vi "Blue to yellow 3.vi"   [LabVIEW 2019]
uses:
  Global Var.vi
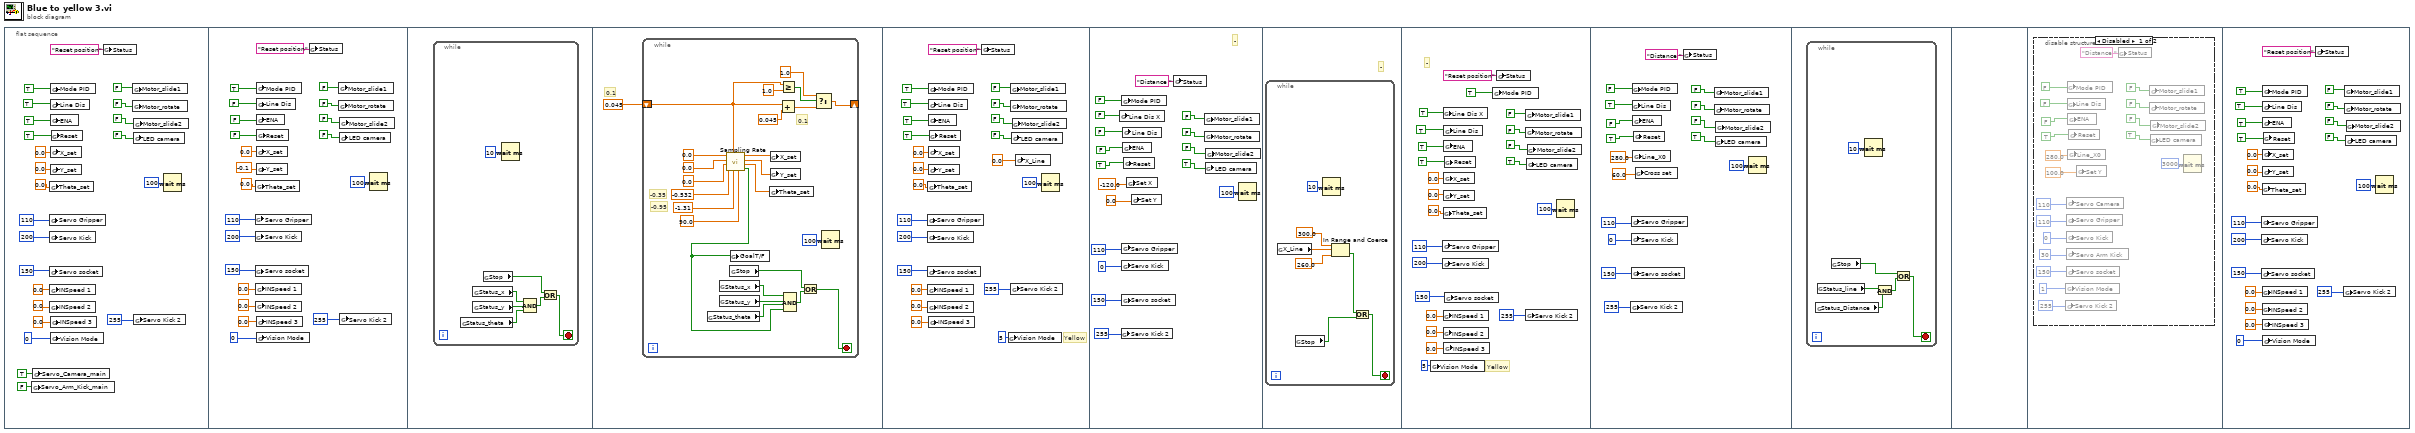
[diagram p0: block diagram]
diagram:
  n1 = flat-sequence {
    frame #0 {
      n2 = global write "Global Var.vi" "Servo_Arm_Kick_main"(FALSE ("Mode PID")) -> ()
      n3 = global write "Global Var.vi" "Servo_Camera_main"(TRUE ("Mode PID")) -> ()
      n4 = global write "Global Var.vi" "Servo Gripper"(u8 110 ("Servo Camera")) -> ()
      n5 = global write "Global Var.vi" "Servo Kick"(u8 200 ("Servo Camera")) -> ()
      n6 = global write "Global Var.vi" "Servo socket"(u8 150 ("Servo Camera")) -> ()
      n7 = global write "Global Var.vi" "Theta_set"(0.0 ("Theta_set")) -> ()
      n8 = global write "Global Var.vi" "INSpeed 1"(0.0 ("X_set")) -> ()
      n9 = global write "Global Var.vi" "INSpeed 2"(0.0 ("Y_set")) -> ()
      n10 = global write "Global Var.vi" "Mode PID"(TRUE ("Mode PID")) -> ()
      n11 = global write "Global Var.vi" "Line Dis"(TRUE ("Mode PID")) -> ()
      n12 = global write "Global Var.vi" "ENA"(TRUE ("ENA")) -> ()
      n13 = global write "Global Var.vi" "X_set"(0.0 ("X_set")) -> ()
      n14 = global write "Global Var.vi" "Y_set"(0.0 ("Y_set")) -> ()
      n15 = global write "Global Var.vi" "INSpeed 3"(0.0 ("Theta_set")) -> ()
      n16 = global write "Global Var.vi" "Vision Mode"(i16 0 ("Vision Mode")) -> ()
      n17 = global write "Global Var.vi" "Reset"(TRUE ("ENA")) -> ()
      n18 = global write "Global Var.vi" "Status"("Reset position" ("Status")) -> ()
      n19 = global write "Global Var.vi" "Motor_slide1"(FALSE ("Mode PID")) -> ()
      n20 = global write "Global Var.vi" "Motor_rotate"(FALSE ("ENA")) -> ()
      n21 = global write "Global Var.vi" "LED camera"(FALSE ("LED camera")) -> ()
      n22 = global write "Global Var.vi" "Motor_slide2"(FALSE ("ENA")) -> ()
      n23 = global write "Global Var.vi" "Servo Kick 2"(u8 255 ("Servo Camera")) -> ()
      n24 = Wait (ms)(milliseconds to wait=u32 100) -> ()  [unwired: 1 out]
    }
    frame #1 {
      n25 = global write "Global Var.vi" "Servo Gripper"(u8 110 ("Servo Camera")) -> ()
      n26 = global write "Global Var.vi" "Servo Kick"(u8 200 ("Servo Camera")) -> ()
      n27 = global write "Global Var.vi" "Servo socket"(u8 150 ("Servo Camera")) -> ()
      n28 = global write "Global Var.vi" "Theta_set"(0.0 ("Theta_set")) -> ()
      n29 = global write "Global Var.vi" "INSpeed 1"(0.0 ("X_set")) -> ()
      n30 = global write "Global Var.vi" "INSpeed 2"(0.0 ("Y_set")) -> ()
      n31 = global write "Global Var.vi" "Mode PID"(TRUE ("Mode PID")) -> ()
      n32 = global write "Global Var.vi" "Line Dis"(FALSE ("Mode PID")) -> ()
      n33 = global write "Global Var.vi" "ENA"(FALSE ("ENA")) -> ()
      n34 = global write "Global Var.vi" "X_set"(0.0 ("X_set")) -> ()
      n35 = global write "Global Var.vi" "Y_set"(-0.1 ("Y_set")) -> ()
      n36 = global write "Global Var.vi" "INSpeed 3"(0.0 ("Theta_set")) -> ()
      n37 = global write "Global Var.vi" "Vision Mode"(i16 0 ("Vision Mode")) -> ()
      n38 = global write "Global Var.vi" "Reset"(FALSE ("ENA")) -> ()
      n39 = global write "Global Var.vi" "Status"("Reset position" ("Status")) -> ()
      n40 = global write "Global Var.vi" "Motor_slide1"(FALSE ("Mode PID")) -> ()
      n41 = global write "Global Var.vi" "Motor_rotate"(FALSE ("ENA")) -> ()
      n42 = global write "Global Var.vi" "LED camera"(FALSE ("LED camera")) -> ()
      n43 = global write "Global Var.vi" "Motor_slide2"(FALSE ("ENA")) -> ()
      n44 = global write "Global Var.vi" "Servo Kick 2"(u8 255 ("Servo Camera")) -> ()
      n45 = Wait (ms)(milliseconds to wait=u32 100) -> ()  [unwired: 1 out]
    }
    frame #2 {
      n46 = while {
        stop <- w47 stop-if-true
        n47 = global read "Global Var.vi" "Status_theta"() -> (w49:bool)
        n48 = global read "Global Var.vi" "Status_x"() -> (w50:bool)
        n49 = global read "Global Var.vi" "Status_y"() -> (w51:bool)
        n50 = global read "Global Var.vi" "Stop"() -> (w45:bool)
        n51 = Wait (ms)(milliseconds to wait=u32 10) -> ()  [unwired: 1 out]
        n52 = Compound Arithmetic op=AND(w50, w51, w49) -> (w46:bool)
        n53 = Or(x=w45, y=w46) -> (x .or. y?=w47:bool)
      }
    }
    frame #3 {
      # "0.1"
      n54 = while {
        shift-right: [w55] -> _
        shift-left: 0.045 -> [w53]
        stop <- w72 stop-if-true
        # "0.1"
        # "-0.95"
        # "-0.35"
        n55 = global read "Global Var.vi" "Status_theta"() -> (w74:bool)
        n56 = global read "Global Var.vi" "Status_x"() -> (w75:bool)
        n57 = global read "Global Var.vi" "Status_y"() -> (w76:bool)
        n58 = call "Sampling Rate.vi"("input a1"=90.0, "input y1"=-1.31, "T(0-1)"=w53, "input x1"=-0.532, "input a0"=0.0, "input y0"=0.0, "input x0"=0.0) -> ("GoalT/F"=w60:bool, "a_output"=w67:dbl, "y_output"=w68:dbl, "x_output"=w69:dbl)  [unwired: 1 in]
        n59 = global read "Global Var.vi" "Stop"() -> (w70:bool)
        n60 = global write "Global Var.vi" "GoalT/F"(w60) -> ()
        n61 = global write "Global Var.vi" "Theta_set"(w67) -> ()
        n62 = global write "Global Var.vi" "X_set"(w69) -> ()
        n63 = global write "Global Var.vi" "Y_set"(w68) -> ()
        n64 = Add(x=w53, y=0.045) -> (x+y=w58:dbl)
        n65 = Greater Or Equal?(x=w53, y=1.0) -> (x >= y?=w57:bool)
        n66 = Compound Arithmetic op=AND(w75, w76, w74, w60) -> (w71:bool)
        n67 = Or(x=w70, y=w71) -> (x .or. y?=w72:bool)
        n68 = Select(t=1.0, s=w57, f=w58) -> (s? t:f=w55:dbl)
        n69 = Wait (ms)(milliseconds to wait=u32 100) -> ()  [unwired: 1 out]
      }
    }
    frame #4 {
      # "Yellow"
      n70 = global write "Global Var.vi" "Servo Gripper"(u8 110 ("Servo Camera")) -> ()
      n71 = global write "Global Var.vi" "Servo Kick"(u8 200 ("Servo Camera")) -> ()
      n72 = global write "Global Var.vi" "Servo socket"(u8 150 ("Servo Camera")) -> ()
      n73 = global write "Global Var.vi" "Theta_set"(0.0 ("Theta_set")) -> ()
      n74 = global write "Global Var.vi" "INSpeed 1"(0.0 ("X_set")) -> ()
      n75 = global write "Global Var.vi" "INSpeed 2"(0.0 ("Y_set")) -> ()
      n76 = global write "Global Var.vi" "Mode PID"(TRUE ("Mode PID")) -> ()
      n77 = global write "Global Var.vi" "Line Dis"(TRUE ("Mode PID")) -> ()
      n78 = global write "Global Var.vi" "ENA"(TRUE ("ENA")) -> ()
      n79 = global write "Global Var.vi" "X_set"(0.0 ("X_set")) -> ()
      n80 = global write "Global Var.vi" "Y_set"(0.0 ("Y_set")) -> ()
      n81 = global write "Global Var.vi" "INSpeed 3"(0.0 ("Theta_set")) -> ()
      n82 = global write "Global Var.vi" "Reset"(TRUE ("ENA")) -> ()
      n83 = global write "Global Var.vi" "Status"("Reset position" ("Status")) -> ()
      n84 = global write "Global Var.vi" "Vision Mode"(i16 5 ("Vision Mode")) -> ()
      n85 = global write "Global Var.vi" "Motor_slide1"(FALSE ("Mode PID")) -> ()
      n86 = global write "Global Var.vi" "Motor_rotate"(FALSE ("ENA")) -> ()
      n87 = global write "Global Var.vi" "Servo Kick 2"(u8 255 ("Servo Camera")) -> ()
      n88 = global write "Global Var.vi" "LED camera"(FALSE ("LED camera")) -> ()
      n89 = global write "Global Var.vi" "Motor_slide2"(FALSE ("ENA")) -> ()
      n90 = global write "Global Var.vi" "X_Line"(0.0 ("X_set")) -> ()
      n91 = Wait (ms)(milliseconds to wait=u32 100) -> ()  [unwired: 1 out]
    }
    frame #5 {
      # "-"
      n92 = global write "Global Var.vi" "Line Dis X"(FALSE ("Mode PID")) -> ()
      n93 = global write "Global Var.vi" "Servo Kick 2"(u8 255 ("Servo Camera")) -> ()
      n94 = global write "Global Var.vi" "Mode PID"(FALSE ("Mode PID")) -> ()
      n95 = global write "Global Var.vi" "Servo Gripper"(u8 110 ("Servo Camera")) -> ()
      n96 = global write "Global Var.vi" "Servo Kick"(u8 0 ("Servo Camera")) -> ()
      n97 = global write "Global Var.vi" "Servo socket"(u8 150 ("Servo Camera")) -> ()
      n98 = global write "Global Var.vi" "Line Dis"(FALSE ("Mode PID")) -> ()
      n99 = global write "Global Var.vi" "ENA"(FALSE ("ENA")) -> ()
      n100 = global write "Global Var.vi" "Reset"(TRUE ("ENA")) -> ()
      n101 = global write "Global Var.vi" "Set X"(-120.0 ("Y_set")) -> ()
      n102 = global write "Global Var.vi" "Set Y"(0.0 ("Y_set")) -> ()
      n103 = global write "Global Var.vi" "Status"("Distance " ("Status")) -> ()
      n104 = global write "Global Var.vi" "Motor_slide1"(FALSE ("Mode PID")) -> ()
      n105 = global write "Global Var.vi" "Motor_rotate"(FALSE ("ENA")) -> ()
      n106 = global write "Global Var.vi" "LED camera"(TRUE ("LED camera")) -> ()
      n107 = global write "Global Var.vi" "Motor_slide2"(FALSE ("ENA")) -> ()
      n108 = Wait (ms)(milliseconds to wait=u32 100) -> ()  [unwired: 1 out]
    }
    frame #6 {
      # "-"
      n109 = while {
        stop <- w121 stop-if-true
        n110 = global read "Global Var.vi" "X_Line"() -> (w119:dbl)
        n111 = global read "Global Var.vi" "Stop"() -> (w120:bool)
        n112 = Wait (ms)(milliseconds to wait=u32 10) -> ()  [unwired: 1 out]
        n113 = In Range and Coerce(upper limit=300.0, x=w119, lower limit=260.0) -> (In Range?=w116:bool)  [unwired: 1 out]
        n114 = Or(x=w116, y=w120) -> (x .or. y?=w121:bool)
      }
    }
    frame #7 {
      # "-"
      # "Yellow"
      n115 = global write "Global Var.vi" "Vision Mode"(i16 5 ("Vision Mode")) -> ()
      n116 = global write "Global Var.vi" "Servo Gripper"(u8 110 ("Servo Camera")) -> ()
      n117 = global write "Global Var.vi" "Servo Kick"(u8 200 ("Servo Camera")) -> ()
      n118 = global write "Global Var.vi" "Line Dis X"(TRUE ("Mode PID")) -> ()
      n119 = global write "Global Var.vi" "Theta_set"(0.0 ("Theta_set")) -> ()
      n120 = global write "Global Var.vi" "INSpeed 1"(0.0 ("X_set")) -> ()
      n121 = global write "Global Var.vi" "INSpeed 2"(0.0 ("Y_set")) -> ()
      n122 = global write "Global Var.vi" "Line Dis"(TRUE ("Mode PID")) -> ()
      n123 = global write "Global Var.vi" "ENA"(TRUE ("ENA")) -> ()
      n124 = global write "Global Var.vi" "X_set"(0.0 ("X_set")) -> ()
      n125 = global write "Global Var.vi" "Y_set"(0.0 ("Y_set")) -> ()
      n126 = global write "Global Var.vi" "INSpeed 3"(0.0 ("Theta_set")) -> ()
      n127 = global write "Global Var.vi" "Reset"(TRUE ("ENA")) -> ()
      n128 = global write "Global Var.vi" "Servo socket"(u8 150 ("Servo Camera")) -> ()
      n129 = global write "Global Var.vi" "Mode PID"(TRUE ("Mode PID")) -> ()
      n130 = global write "Global Var.vi" "Status"("Reset position" ("Status")) -> ()
      n131 = global write "Global Var.vi" "Motor_slide1"(FALSE ("Mode PID")) -> ()
      n132 = global write "Global Var.vi" "Motor_rotate"(FALSE ("ENA")) -> ()
      n133 = global write "Global Var.vi" "Servo Kick 2"(u8 255 ("Servo Camera")) -> ()
      n134 = global write "Global Var.vi" "LED camera"(TRUE ("LED camera")) -> ()
      n135 = global write "Global Var.vi" "Motor_slide2"(FALSE ("ENA")) -> ()
      n136 = Wait (ms)(milliseconds to wait=u32 100) -> ()  [unwired: 1 out]
    }
    frame #8 {
      n137 = global write "Global Var.vi" "Servo Kick 2"(u8 255 ("Servo Camera")) -> ()
      n138 = global write "Global Var.vi" "Servo Gripper"(u8 110 ("Servo Camera")) -> ()
      n139 = global write "Global Var.vi" "Servo Kick"(u8 0 ("Servo Camera")) -> ()
      n140 = global write "Global Var.vi" "Servo socket"(u8 150 ("Servo Camera")) -> ()
      n141 = global write "Global Var.vi" "Mode PID"(FALSE ("Mode PID")) -> ()
      n142 = global write "Global Var.vi" "Line Dis"(TRUE ("Mode PID")) -> ()
      n143 = global write "Global Var.vi" "ENA"(FALSE ("ENA")) -> ()
      n144 = global write "Global Var.vi" "Line_X0"(280.0 ("Y_set")) -> ()
      n145 = global write "Global Var.vi" "Reset"(TRUE ("ENA")) -> ()
      n146 = global write "Global Var.vi" "Cross set"(60.0 ("Y_set")) -> ()
      n147 = global write "Global Var.vi" "Status"("Distance " ("Status")) -> ()
      n148 = global write "Global Var.vi" "Motor_slide1"(FALSE ("Mode PID")) -> ()
      n149 = global write "Global Var.vi" "Motor_rotate"(FALSE ("ENA")) -> ()
      n150 = global write "Global Var.vi" "LED camera"(TRUE ("LED camera")) -> ()
      n151 = global write "Global Var.vi" "Motor_slide2"(FALSE ("ENA")) -> ()
      n152 = Wait (ms)(milliseconds to wait=u32 100) -> ()  [unwired: 1 out]
    }
    frame #9 {
      n153 = while {
        stop <- w165 stop-if-true
        n154 = global read "Global Var.vi" "Status_Distance"() -> (w161:bool)
        n155 = global read "Global Var.vi" "Status_line"() -> (w162:bool)
        n156 = global read "Global Var.vi" "Stop"() -> (w164:bool)
        n157 = Wait (ms)(milliseconds to wait=u32 10) -> ()  [unwired: 1 out]
        n158 = And(x=w162, y=w161) -> (x .and. y?=w163:bool)
        n159 = Or(x=w164, y=w163) -> (x .or. y?=w165:bool)
      }
    }
    frame #10 {
    }
    frame #11 {
      n160 = disable-structure shown="Disabled" {
        frame Disabled {
          n161 = global write "Global Var.vi" "Servo Kick 2"(u8 255 ("Servo Camera")) -> ()
          n162 = global write "Global Var.vi" "Vision Mode"(i16 1 ("Vision Mode")) -> ()
          n163 = global write "Global Var.vi" "Servo Camera"(u8 110 ("Servo Camera")) -> ()
          n164 = global write "Global Var.vi" "Servo Gripper"(u8 110 ("Servo Camera")) -> ()
          n165 = global write "Global Var.vi" "Servo Kick"(u8 0 ("Servo Camera")) -> ()
          n166 = global write "Global Var.vi" "Servo Arm Kick"(u8 30 ("Servo Camera")) -> ()
          n167 = global write "Global Var.vi" "Servo socket"(u8 150 ("Servo Camera")) -> ()
          n168 = global write "Global Var.vi" "Mode PID"(FALSE ("Mode PID")) -> ()
          n169 = global write "Global Var.vi" "Line Dis"(FALSE ("Mode PID")) -> ()
          n170 = global write "Global Var.vi" "ENA"(FALSE ("ENA")) -> ()
          n171 = global write "Global Var.vi" "Line_X0"(280.0 ("Y_set")) -> ()
          n172 = global write "Global Var.vi" "Reset"(TRUE ("ENA")) -> ()
          n173 = global write "Global Var.vi" "Set Y"(100.0 ("Y_set")) -> ()
          n174 = global write "Global Var.vi" "Status"("Distance " ("Status")) -> ()
          n175 = global write "Global Var.vi" "Motor_slide1"(FALSE ("Mode PID")) -> ()
          n176 = global write "Global Var.vi" "Motor_rotate"(FALSE ("ENA")) -> ()
          n177 = global write "Global Var.vi" "LED camera"(TRUE ("LED camera")) -> ()
          n178 = global write "Global Var.vi" "Motor_slide2"(FALSE ("ENA")) -> ()
          n179 = Wait (ms)(milliseconds to wait=u32 3000) -> ()  [unwired: 1 out]
        }
        frame Enabled {
        }
      }
    }
    frame #12 {
      n180 = global write "Global Var.vi" "Servo Gripper"(u8 110 ("Servo Camera")) -> ()
      n181 = global write "Global Var.vi" "Servo Kick"(u8 200 ("Servo Camera")) -> ()
      n182 = global write "Global Var.vi" "Servo socket"(u8 150 ("Servo Camera")) -> ()
      n183 = global write "Global Var.vi" "Theta_set"(0.0 ("Theta_set")) -> ()
      n184 = global write "Global Var.vi" "INSpeed 1"(0.0 ("X_set")) -> ()
      n185 = global write "Global Var.vi" "INSpeed 2"(0.0 ("Y_set")) -> ()
      n186 = global write "Global Var.vi" "Mode PID"(TRUE ("Mode PID")) -> ()
      n187 = global write "Global Var.vi" "Line Dis"(TRUE ("Mode PID")) -> ()
      n188 = global write "Global Var.vi" "ENA"(TRUE ("ENA")) -> ()
      n189 = global write "Global Var.vi" "X_set"(0.0 ("X_set")) -> ()
      n190 = global write "Global Var.vi" "Y_set"(0.0 ("Y_set")) -> ()
      n191 = global write "Global Var.vi" "INSpeed 3"(0.0 ("Theta_set")) -> ()
      n192 = global write "Global Var.vi" "Vision Mode"(i16 0 ("Vision Mode")) -> ()
      n193 = global write "Global Var.vi" "Reset"(TRUE ("ENA")) -> ()
      n194 = global write "Global Var.vi" "Status"("Reset position" ("Status")) -> ()
      n195 = global write "Global Var.vi" "Servo Kick 2"(u8 255 ("Servo Camera")) -> ()
      n196 = global write "Global Var.vi" "Motor_slide1"(FALSE ("Mode PID")) -> ()
      n197 = global write "Global Var.vi" "Motor_rotate"(FALSE ("ENA")) -> ()
      n198 = global write "Global Var.vi" "LED camera"(FALSE ("LED camera")) -> ()
      n199 = global write "Global Var.vi" "Motor_slide2"(FALSE ("ENA")) -> ()
      n200 = Wait (ms)(milliseconds to wait=u32 100) -> ()  [unwired: 1 out]
    }
  }
